vi "Table Control_1D.vi"(0 "CtlRef":refnum<vi>, 1 "Header Row(F)/Column(T)":bool, 2 "Valid Indexes":i32[](array[numeric]), 5 "CharIn":i16, 7 "VKey":T1, 9 "ScanCode":i16) -> (6 "CharOut":i16, 15 "Discard?":bool)   [LabVIEW 2013]
uses:
  <vilib>/event_ctls.llb/eventvkey.ctl
  <vilib>/Utility/miscctls.llb/LVRowAndColumnTypeDef.ctl
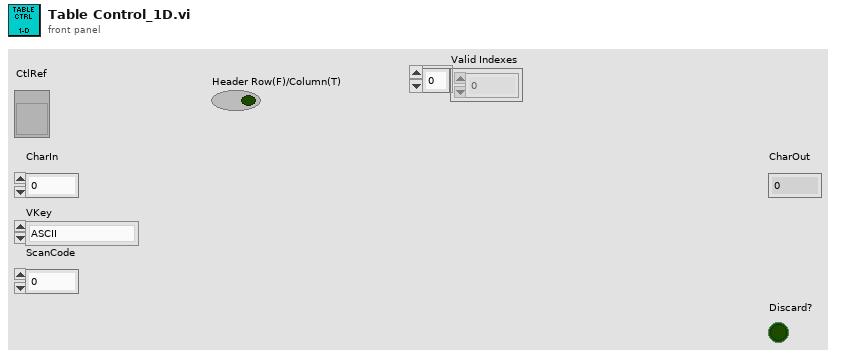
[diagram p1: front panel]
types:
  T1 = typedef "eventvkey.ctl" = enum16{"ASCII", "Enter", "Return", "Shift", "Ctrl", "Alt", "Cmd", "Opt", "Caps", "NumLock", "Clear", "Break", "Up", "Down", "Left", "Right", "Insert", "Delete", "Home", "End", "PageUp", "PageDown", "Escape", "Help", "Pause", "ScrollLock", "F1", "F2", "F3", "F4", "F5", "F6", "F7", "F8", "F9", "F10", "F11", "F12", "F13", "F14", "F15", "F16", "F17", "F18", "F19", "F20", "F21", "F22", "F23", "F24", "Play", "VolumeUp", "VolumeDown", "Mute", "Two Byte Char"}
  T2 = typedef "LVRowAndColumnTypeDef.ctl" = cluster{"Row":i32, "Column":i32}
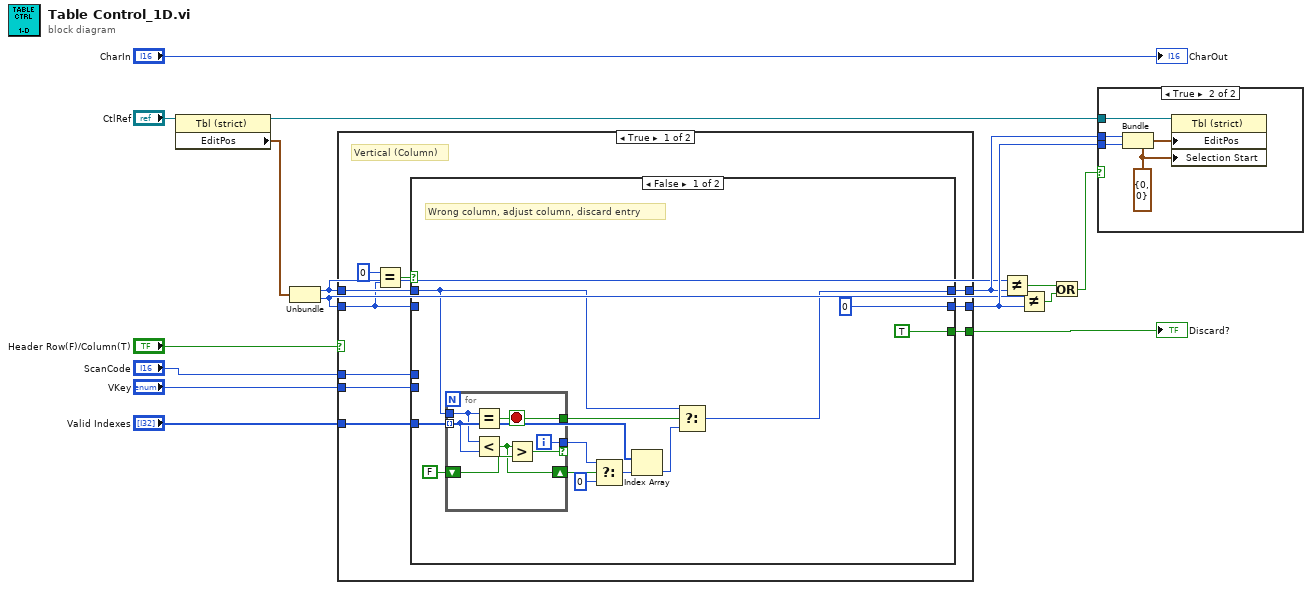
[diagram p0: block diagram]
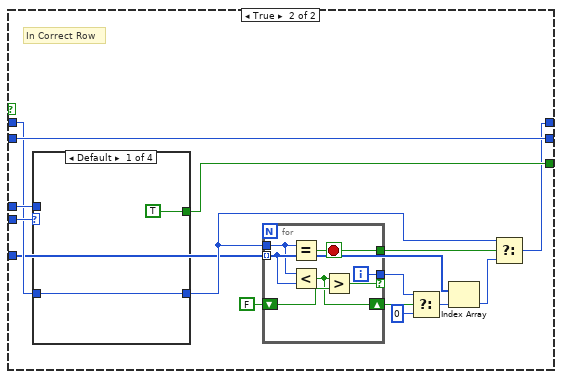
[diagram p3: hidden frame]
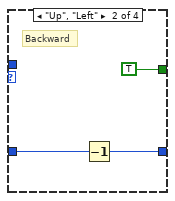
[diagram p4: hidden frame]
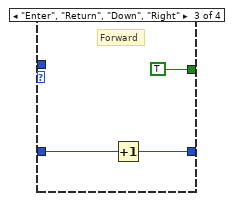
[diagram p5: hidden frame]
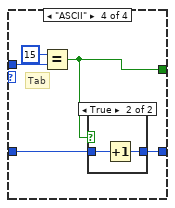
[diagram p6: hidden frame]
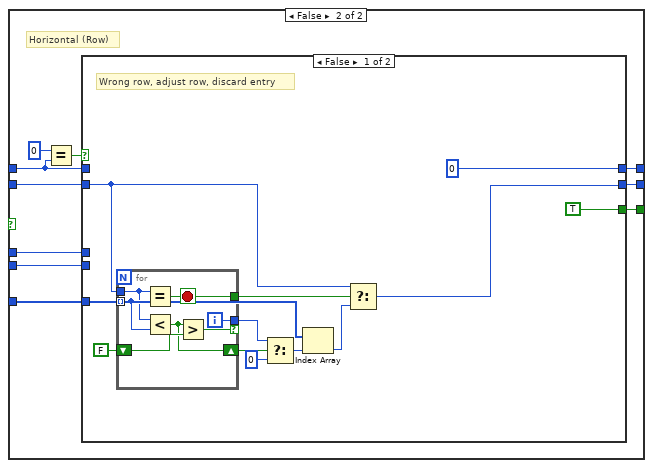
[diagram p8: hidden frame]
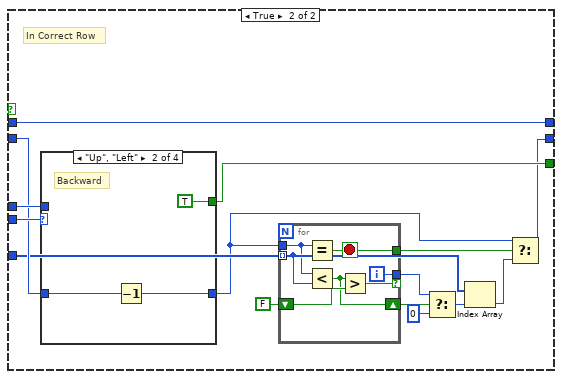
[diagram p9: hidden frame]
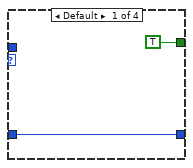
[diagram p10: hidden frame]
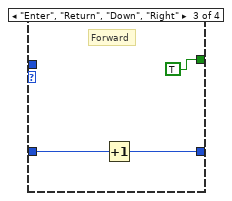
[diagram p11: hidden frame]
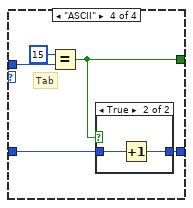
[diagram p12: hidden frame]
diagram:
  n1 = property on="Property Node" class="Tbl (strict)"(reference="CtlRef") -> (reference out=w15:refnum<vi>, "EditPos"=w13:T2)  [unwired: 1 in, 1 out]
  n2 = Unbundle(w13) -> ("Row"=w4:i32, "Column"=w6:i32)
  n3 = case shown="True" "Header Row(F)/Column(T)" {
    tunnel: w4 -> [w26 w87]
    tunnel: w6 -> [w18 w91]
    tunnel: "Valid Indexes" -> [w20 w90]
    tunnel: [w25 w89] -> w5
    tunnel: [w24 w88] -> w7
    tunnel: [w23 w86] -> w8
    tunnel: "ScanCode" -> [w22 w85]
    tunnel: "VKey" -> [w21 w84]
    frame True {
      # "Vertical (Column)"
      n4 = Equal?(x=0, y=w18) -> (x = y?=w17:bool)
      n5 = case shown="False" w17 {
        tunnel: w18 -> [_ w57]
        tunnel: w20 -> [w32 w46]
        tunnel: [w28 w47] -> w25
        tunnel: [0 w57] -> w24
        tunnel: w26 -> [w29 w56]
        tunnel: [TRUE w58] -> w23
        tunnel: w22 -> [_ w60]
        tunnel: w21 -> [_ w59]
        frame False {
          # "Wrong column, adjust column, discard entry"
          n6 = for {
            tunnel: w32 -> [w43] mode=indexing
            tunnel: w29 -> [w44]
            tunnel: [w45] -> w38
            shift-right: [w39] -> w36
            shift-left: FALSE -> [w42]
            tunnel: [w41] -> w35 if=w40
            i -> [w41]
            stop <- w45 stop-if-true
            n7 = Equal?(x=w44, y=w43) -> (x = y?=w45:bool)
            n8 = Less?(x=w44, y=w43) -> (x < y?=w39:bool)
            n9 = Greater?(x=w39, y=w42) -> (0:w40:bool)
          }
          n10 = Select(t=w35, s=w36, f=0) -> (s? t:f=w33:i32)
          n11 = Index Array(array=w32, index=w33) -> (element=w31:i32)
          n12 = Select(t=w29, s=w38, f=w31) -> (s? t:f=w28:i32)
        }
        frame True {
          # "In Correct Row"
          n13 = case shown="Default" w59 {
            tunnel: w60 -> [_ _ _ w79]
            tunnel: w56 -> [w69 w71 w74 w78]
            tunnel: [w69 w70 w73 w77] -> w48
            tunnel: [TRUE TRUE TRUE w76] -> w58
            frame Default {
            }
            frame "Up", "Left" {
              # "Backward"
              n14 = Decrement(x=w71) -> (x-1=w70:i32)
            }
            frame "Enter", "Return", "Down", "Right" {
              # "Forward"
              n15 = Increment(x=w74) -> (x+1=w73:i32)
            }
            frame "ASCII" {
              # "Tab"
              n16 = Equal?(x=i16 15, y=w79) -> (x = y?=w76:bool)
              n17 = case shown="True" w76 {
                tunnel: w78 -> [w81 w83]
                tunnel: [w81 w82] -> w77
                frame False {
                }
                frame True {
                  n18 = Increment(x=w83) -> (x+1=w82:i32)
                }
              }
            }
          }
          n19 = for {
            tunnel: w46 -> [w65] mode=indexing
            tunnel: w48 -> [w66]
            tunnel: [w67] -> w55
            shift-right: [w61] -> w53
            shift-left: FALSE -> [w64]
            tunnel: [w63] -> w52 if=w62
            i -> [w63]
            stop <- w67 stop-if-true
            n20 = Equal?(x=w66, y=w65) -> (x = y?=w67:bool)
            n21 = Less?(x=w66, y=w65) -> (x < y?=w61:bool)
            n22 = Greater?(x=w61, y=w64) -> (0:w62:bool)
          }
          n23 = Select(t=w52, s=w53, f=0) -> (s? t:f=w50:i32)
          n24 = Index Array(array=w46, index=w50) -> (element=w49:i32)
          n25 = Select(t=w48, s=w55, f=w49) -> (s? t:f=w47:i32)
        }
      }
    }
    frame False {
      # "Horizontal (Row)"
      n26 = Equal?(x=0, y=w87) -> (x = y?=w92:bool)
      n27 = case shown="False" w92 {
        tunnel: w91 -> [w96 w124]
        tunnel: w90 -> [w98 w114]
        tunnel: [0 w127] -> w89
        tunnel: [w95 w115] -> w88
        tunnel: w87 -> [_ w127]
        tunnel: [TRUE w123] -> w86
        tunnel: w85 -> [_ w126]
        tunnel: w84 -> [_ w125]
        frame False {
          # "Wrong row, adjust row, discard entry"
          n28 = for {
            tunnel: w98 -> [w110] mode=indexing
            tunnel: w96 -> [w111]
            tunnel: [w112] -> w104
            shift-right: [w106] -> w102
            shift-left: FALSE -> [w109]
            tunnel: [w108] -> w101 if=w107
            i -> [w108]
            stop <- w112 stop-if-true
            n29 = Equal?(x=w111, y=w110) -> (x = y?=w112:bool)
            n30 = Less?(x=w111, y=w110) -> (x < y?=w106:bool)
            n31 = Greater?(x=w106, y=w109) -> (0:w107:bool)
          }
          n32 = Select(t=w101, s=w102, f=0) -> (s? t:f=w99:i32)
          n33 = Index Array(array=w98, index=w99) -> (element=w97:i32)
          n34 = Select(t=w96, s=w104, f=w97) -> (s? t:f=w95:i32)
        }
        frame True {
          # "In Correct Row"
          n35 = case shown="\"Up\", \"Left\"" w125 {
            tunnel: w126 -> [_ _ _ w146]
            tunnel: w124 -> [w136 w138 w141 w145]
            tunnel: [w136 w137 w140 w144] -> w113
            tunnel: [TRUE TRUE TRUE w143] -> w123
            frame Default {
            }
            frame "Up", "Left" {
              # "Backward"
              n36 = Decrement(x=w138) -> (x-1=w137:i32)
            }
            frame "Enter", "Return", "Down", "Right" {
              # "Forward"
              n37 = Increment(x=w141) -> (x+1=w140:i32)
            }
            frame "ASCII" {
              # "Tab"
              n38 = Equal?(x=i16 15, y=w146) -> (x = y?=w143:bool)
              n39 = case shown="True" w143 {
                tunnel: w145 -> [w148 w150]
                tunnel: [w148 w149] -> w144
                frame False {
                }
                frame True {
                  n40 = Increment(x=w150) -> (x+1=w149:i32)
                }
              }
            }
          }
          n41 = for {
            tunnel: w114 -> [w132] mode=indexing
            tunnel: w113 -> [w133]
            tunnel: [w134] -> w122
            shift-right: [w128] -> w120
            shift-left: FALSE -> [w131]
            tunnel: [w130] -> w119 if=w129
            i -> [w130]
            stop <- w134 stop-if-true
            n42 = Equal?(x=w133, y=w132) -> (x = y?=w134:bool)
            n43 = Less?(x=w133, y=w132) -> (x < y?=w128:bool)
            n44 = Greater?(x=w128, y=w131) -> (0:w129:bool)
          }
          n45 = Select(t=w119, s=w120, f=0) -> (s? t:f=w117:i32)
          n46 = Index Array(array=w114, index=w117) -> (element=w116:i32)
          n47 = Select(t=w113, s=w122, f=w116) -> (s? t:f=w115:i32)
        }
      }
    }
  }
  "Discard?" <- w8
  n48 = Not Equal?(x=w4, y=w5) -> (x != y?=w3:bool)
  n49 = Not Equal?(x=w6, y=w7) -> (x != y?=w2:bool)
  n50 = Or(x=w3, y=w2) -> (x .or. y?=w1:bool)
  n51 = case shown="True" w1 {
    tunnel: w15 -> [_ w155]
    tunnel: w7 -> [_ w152]
    tunnel: w5 -> [_ w151]
    frame False {
    }
    frame True {
      w153 = T2 {"Row"=0, "Column"=0} ("Active Cell:Active Cell")
      n52 = Bundle(cluster=w153, "Row"=w151, "Column"=w152) -> (w154:T2)
      n53 = property on="Property Node" class="Tbl (strict)"(reference=w155, "EditPos"=w154, "Selection Start"=w153) -> ()  [unwired: 1 in, 2 out]
    }
  }
  "CharOut" <- "CharIn"
